vi "Log Command Message.vi"(5 "Level":T1, 6 "Command Message":refnum<class "Command Message Interface.lvclass">, 7 "Actor":refnum<class "Ancestral Actor.lvclass">, 8 "error in (no error)":errorcluster, 11 "Application Log in":refnum<class "Application Log.lvclass">) -> (0 "error out":errorcluster, 3 "Application Log out":refnum<class "Application Log.lvclass">)   [LabVIEW 2016, in "Stream Log.lvlib" / "Application Log.lvclass"]
doc: "--\nCopyright © 2017 Composed SystemsI All rights reserved.\n\nAuthor: Jon McBee <jon.mcbee@composed.io>\n\nThis library is provided \"AS IS\" ,WITHOUT WARRANTIES OR\nCONDITIONS OF ANY KIND, either express or implied.\n\nComposed Systems -- composed.io\n\nStream 0.0.1.1\nJon McBee - Composed Systems\nCopyright (c) 2017, Composed Systems"
uses:
  <userlib>/Composed Systems/Stream/Log/Application Log/Application Log.lvclass
  <userlib>/Composed Systems/Stream/Log/Application Log/Log Level.ctl
  <userlib>/Composed Systems/Stream/Mediator/Classes/Message Command Interface/Command Message Interface.lvclass
  C:/Program Files (x86)/National Instruments/LabVIEW 2016/user.lib/Composed Systems/Stream/Mediator/Classes/Message Interface/Message Interface.lvclass
  <userlib>/Composed Systems/Stream/Actor/Actor Class/Ancestral Actor.lvclass
  <userlib>/Composed Systems/Stream/Actor/Actor Class/Ancestral Actor.lvclass/Ancestral Actor.ctl
  <userlib>/Composed Systems/Stream/Mediator/Classes/Message Command Interface/Command Message Interface.lvclass/Command Message Interface.ctl
  <userlib>/Composed Systems/Stream/Mediator/Classes/Message Interface/Message Interface.lvclass
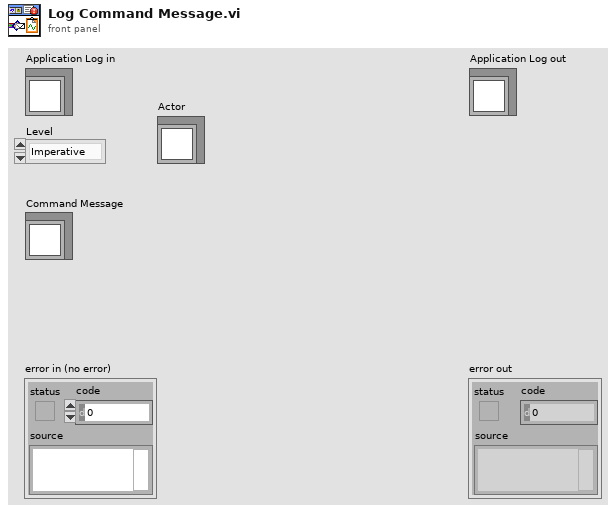
[diagram p1: front panel]
types:
  T1 = typedef "Stream Log.lvlib/Application Log.lvclass/Log Level.ctl" = enum16{"Imperative", "Major", "Minor", "Debug", "Off"}
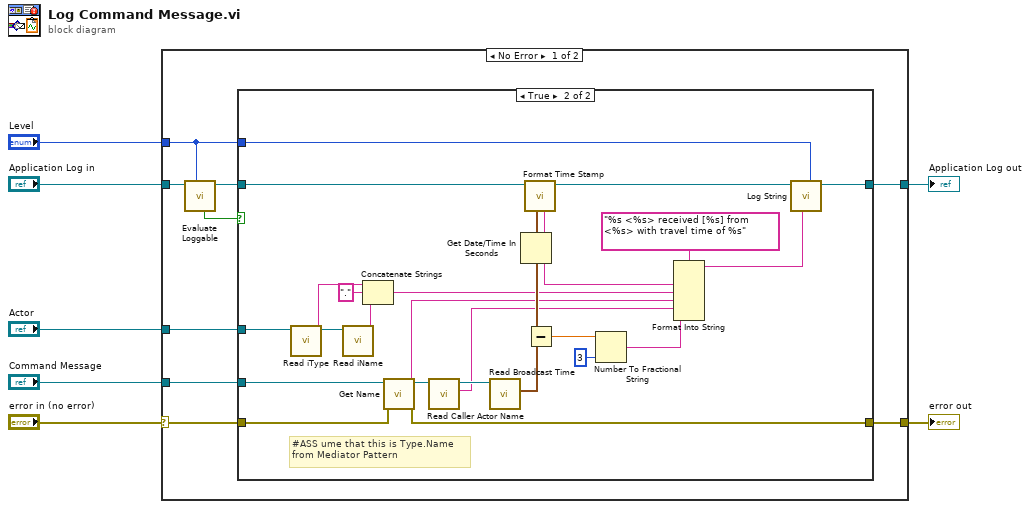
[diagram p0: block diagram]
diagram:
  n1 = case shown="No Error" "error in (no error)" {
    selector: "error in (no error)" -> [w14 w45]
    tunnel: [w10 w45] -> w6
    tunnel: [w12 w44] -> w4
    tunnel: "Application Log in" -> [w16 w44]
    tunnel: "Level" -> [w9 _]
    tunnel: "Command Message" -> [w15 _]
    tunnel: "Actor" -> [w8 _]
    frame No Error {
      n2 = call <userlib>:"Evaluate Loggable.vi"("Level"=w9, "Application Log in"=w16) -> ("Application Log out"=w13:refnum<class "Application Log.lvclass">, "Log?"=w11:bool)  [unwired: 8 in]
      n3 = case shown="True" w11 {
        tunnel: w15 -> [_ w29]
        tunnel: w14 -> [w18 w30]
        tunnel: w13 -> [w17 w41]
        tunnel: [w17 w43] -> w12
        tunnel: [w18 w21] -> w10
        tunnel: w9 -> [_ w42]
        tunnel: w8 -> [_ w27]
        frame False {
        }
        frame True {
          # "#ASS ume that this is Type.Name\nfrom Mediator Pattern"
          n4 = call <userlib>:"Read iType.vi"("Ancestral Actor in"=w27) -> ("iType"=w25:string, "Ancestral Actor out"=w26:refnum<class "Ancestral Actor.lvclass">)  [unwired: 8 in, 1 out]
          n5 = call <userlib>:"Read iName.vi"("Ancestral Actor in"=w26) -> ("iName"=w24:string)  [unwired: 8 in, 2 out]
          n6 = Concatenate Strings(w25, "." ("string"), w24) -> (w35:string)
          n7 = call <userlib>:"Get Name.vi"("error in (no error)"=w30, "Message Interface in"=w29) -> ("error out"=w21:errorcluster, "Name"=w28:string, "Message Interface out"=w23:refnum<class "Command Message Interface.lvclass">)  [unwired: 7 in]
          n8 = call <userlib>:"Read Caller Actor Name.vi"("Command Message Interface in"=w23) -> ("Caller Actor Name"=w20:string, "Command Message Interface out"=w22:refnum<class "Command Message Interface.lvclass">)  [unwired: 9 in]
          n9 = call <userlib>:"Read Broadcast Time.vi"("Command Message Interface in"=w22) -> ("Broadcast Time"=w19:timestamp)  [unwired: 9 in, 1 out]
          n10 = Get Date/Time In Seconds() -> (seconds since 1Jan1904=w38:timestamp)
          n11 = call <userlib>:"Format Time Stamp.vi"("Time Stamp"=w38, "Application Log in"=w41) -> ("Application Log out"=w40:refnum<class "Application Log.lvclass">, "Formatted Time Stamp"=w37:string)  [unwired: 7 in, 1 out]
          n12 = Subtract(x=w19, y=w38) -> (x-y=w34:dbl)
          n13 = Number To Fractional String(number=w34, precision (6)=i16 3) -> (F-format string=w32:string)  [unwired: 2 in]
          n14 = Format Into String(format string="%s <%s> received [%s] from <%s> with travel time of %s", w37, w35, w28, w20, w32) -> (resulting string=w31:string)  [unwired: 2 in, 1 out]
          n15 = call-dynamic "Log String.vi"("Level"=w42, "String"=w31, "Application Log in"=w40) -> ("Application Log out"=w43:refnum<class "Application Log.lvclass">)  [unwired: 7 in, 1 out]
        }
      }
    }
    frame Error {
    }
  }
  "error out" <- w6
  "Application Log out" <- w4
